vi "GFITS_LibWriteHdrs.vi"(7 "file ref":u64, 8 "error in (no error)":errorcluster, 9 "dnum":i32, 10 "Table In":string[][](table), 11 "data type":i32[](array[numeric])) -> (0 "error out":errorcluster)   [LabVIEW 2016]
uses:
  c/lib/libgfits.so
panel:
  out "output param":i32
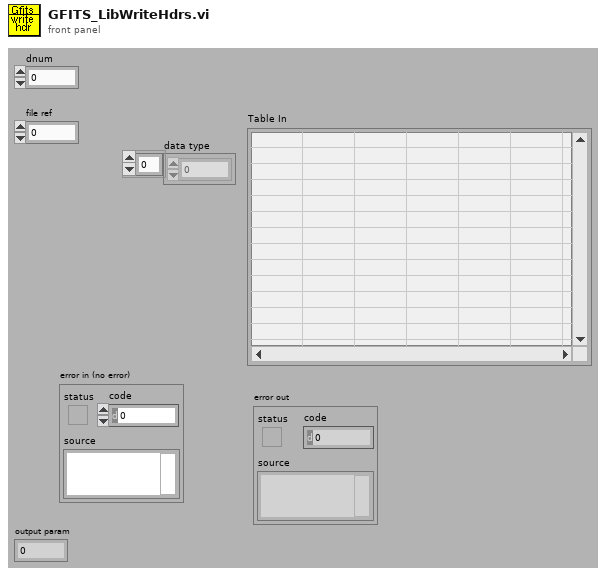
[diagram p1: front panel]
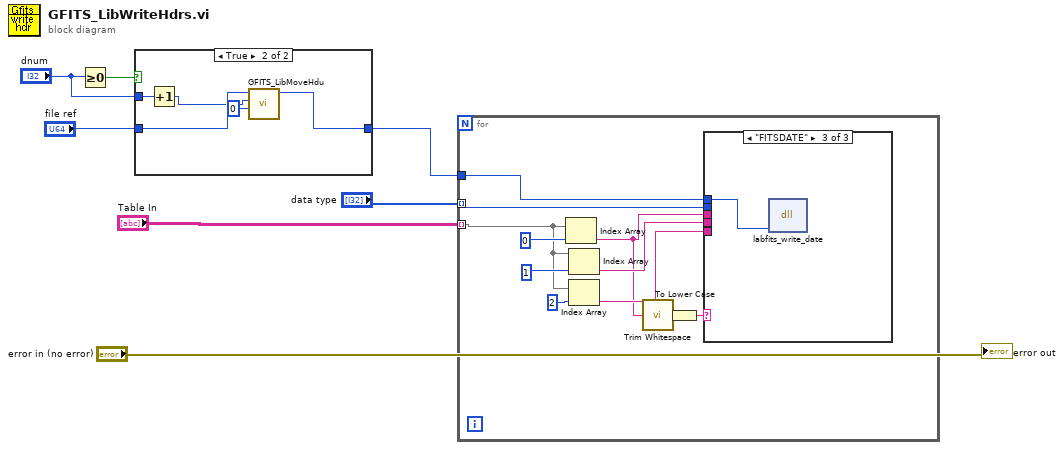
[diagram p0: block diagram]
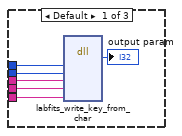
[diagram p3: hidden frame]
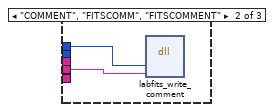
[diagram p4: hidden frame]
diagram:
  n1 = Greater Or Equal To 0?(x="dnum") -> (x >= 0?=w4:bool)
  n2 = case shown="True" w4 {
    tunnel: "file ref" -> [w8 w12]
    tunnel: [w8 w9] -> w2
    tunnel: "dnum" -> [_ w13]
    frame False {
    }
    frame True {
      n3 = Increment(x=w13) -> (x+1=w11:i32)
      n4 = call "GFITS_LibMoveHdu.vi"("hdutype"=0, "hdunum"=w11, "ref"=w12) -> ("ref out"=w9:u64)  [unwired: 1 in, 7 out]
    }
  }
  n5 = for {
    tunnel: "data type" -> [w20] mode=indexing
    tunnel: "Table In" -> [w19] mode=indexing
    tunnel: w2 -> [w21]
    n6 = Index Array(array=w19, index=0) -> (element=w14:string)
    n7 = Index Array(array=w19, index=1) -> (element=w17:string)
    n8 = Index Array(array=w19, index=2) -> (element=w18:string)
    n9 = call <vilib>:"Trim Whitespace.vi"("string"=w14) -> ("trimmed string"=w16:string)  [unwired: 1 in]
    n10 = To Lower Case(string=w16) -> (all lower case string=w15:string)
    n11 = case shown="\"FITSDATE\"" w15 {
      tunnel: w21 -> [w29 w32 w33]
      tunnel: w20 -> [w28 _ _]
      tunnel: w14 -> [w27 _ _]
      tunnel: w17 -> [w26 w31 _]
      tunnel: w18 -> [w25 _ _]
      frame Default {
        n12 = dll-call lib="home/simager/panview/PAN/Modules/GFITS/private/c/lib/libgfits.so" fn="labfits_write_key_from_char" ("libdhs.so:DHS_write_key_from_char")("ref"=w29, "datatype"=w28, "keyname"=w27, "value"=w26, "comment"=w25) -> ("return type"=→"output param":i32)  [unwired: 8 in, 2 out]
      }
      frame "COMMENT", "FITSCOMM", "FITSCOMMENT" {
        n13 = dll-call lib="home/simager/panview/PAN/Modules/GFITS/private/c/lib/libgfits.so" fn="labfits_write_comment" ("libdhs.so:DHS_write_comment")("ref"=w32, "comment"=w31) -> ()  [unwired: 5 in, 3 out]
      }
      frame "FITSDATE" {
        n14 = dll-call lib="home/simager/panview/PAN/Modules/GFITS/private/c/lib/libgfits.so" fn="labfits_write_date" ("libdhs.so:DHS_write_date")("ref"=w33) -> ()  [unwired: 4 in, 3 out]
      }
    }
  }
  "error out" <- "error in (no error)"
